vi "Start Test.vi"(8 "error in (no error)":errorcluster, 10 "Tests":string[](array[string]), 11 "Result Model In":refnum<class "Result Model by Reference.lvclass">) -> (0 "error out":errorcluster)   [LabVIEW 2020, in "Result Model by Reference.lvclass"]
uses:
  Result Model by Reference.lvclass
  Result Model by Reference.lvclass/Result Model by Reference.ctl
  Result Model/Result Model.lvclass
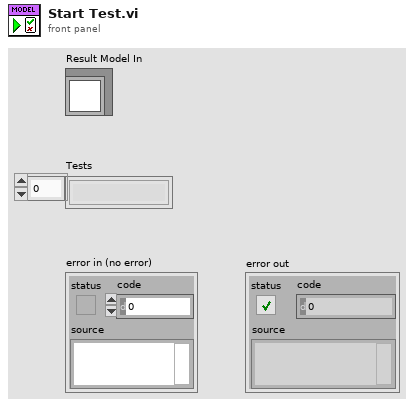
[diagram p1: front panel]
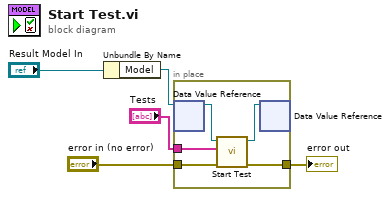
[diagram p0: block diagram]
diagram:
  n1 = Unbundle By Name("Result Model In") -> ("Model"=w4:refnum<data-value>)
  n2 = in-place {
    in-place-border: "error in (no error)" -> [w10]
    in-place-border: [w9] -> w2
    in-place-border: "Tests" -> [w6]
    n3 = in-place-dvr #1(w4) -> (w7:refnum<class "Result Model.lvclass">)  [unwired: 1 out]
    n4 = call "Start Test.vi"("error in (no error)"=w10, "Tests"=w6, "Result Model In"=w7) -> ("error out"=w9:errorcluster, "Result Model Out"=w8:refnum<class "Result Model.lvclass">)  [unwired: 7 in]
    n5 = in-place-dvr #1(w8) -> ()  [unwired: 2 out]
  }
  "error out" <- w2
